vi "Simple QMH Template.vi"   [LabVIEW 2020, in "Volatus.lvlib"]
uses:
  Volatus.lvlib
  Module/Module.lvclass
types:
  T1 = enum32{"Invalid", "Standard", "Closed", "Hidden", "Minimized", "Maximized"}
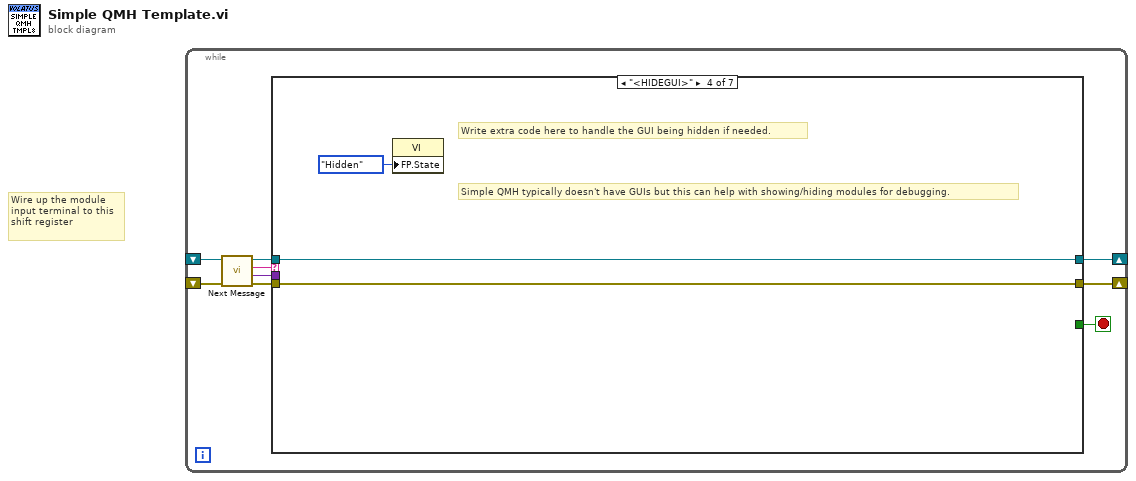
[diagram p0: block diagram]
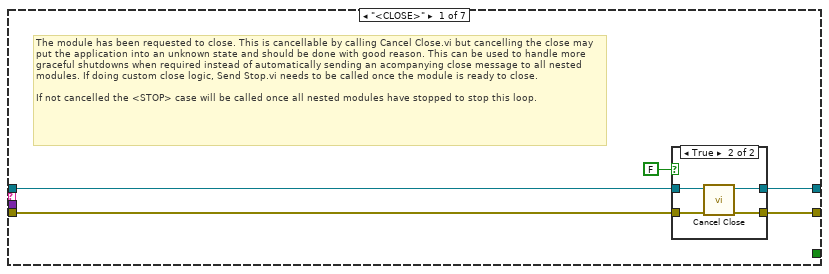
[diagram p2: hidden frame]
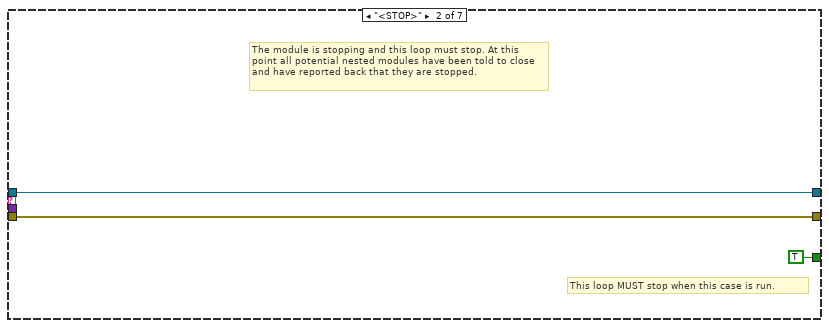
[diagram p4: hidden frame]
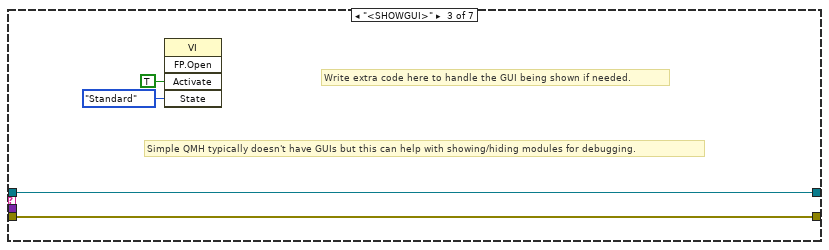
[diagram p5: hidden frame]
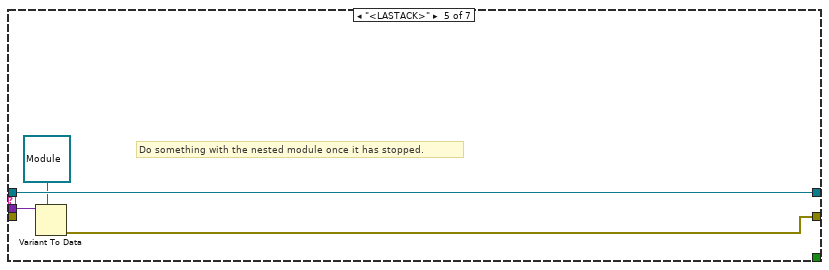
[diagram p6: hidden frame]
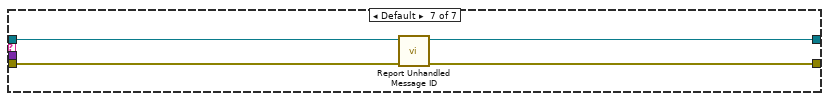
[diagram p8: hidden frame]
diagram:
  # "Wire up the module input terminal to this shift register"
  n1 = while {
    shift-right: [w4] -> _
    shift-left: _ -> [w9]
    shift-right: [w3] -> _
    shift-left: _ -> [w8]
    stop <- w2 stop-if-true
    n2 = call "Next Message.vi"("error in (no error)"=w8, "Module in"=w9) -> ("error out"=w7:errorcluster, "Data"=w1:variant, "ID"=w6:string, "Module out"=w5:refnum<class "Module.lvclass">)  [unwired: 6 in]
    n3 = case shown="\"<HIDEGUI>\"" w6 {
      tunnel: w7 -> [w14 w22 w26 w29 _ w35 w40]
      tunnel: w5 -> [w12 w23 w27 w30 w34 w36 w38]
      tunnel: [w11 w23 w27 w30 w34 w36 w37] -> w4
      tunnel: [w13 w22 w26 w29 w31 w35 w39] -> w3
      tunnel: [_ TRUE _ _ _ _ _] -> w2
      tunnel: w1 -> [_ _ _ _ w33 _ _]
      frame "<CLOSE>" {
        # "The module has been requested to close. This is cancellable by calling Cancel Close.vi but cancelling the close may put the application into an unknown state and should be done with good reason. This can be used to handle more graceful shutdowns when required instead of automatically sending an acompanying close message to all nested modules. If doing custom close logic, Send Stop.vi needs to be called once the module is ready to close.\n\nIf not cancelled the <STOP> case will be called once all nested modules have stopped to stop this loop."
        n4 = case shown="True" FALSE {
          tunnel: w14 -> [w15 w20]
          tunnel: [w15 w19] -> w13
          tunnel: w12 -> [w16 w18]
          tunnel: [w16 w17] -> w11
          frame False {
          }
          frame True {
            n5 = call "Cancel Close.vi"("error in (no error)"=w20, "Module in"=w18) -> ("error out"=w19:errorcluster, "Module out"=w17:refnum<class "Module.lvclass">)  [unwired: 8 in]
          }
        }
      }
      frame "<STOP>" {
        # "This loop MUST stop when this case is run."
        # "The module is stopping and this loop must stop. At this point all potential nested modules have been told to close and have reported back that they are stopped."
      }
      frame "<SHOWGUI>" {
        # "Simple QMH typically doesn't have GUIs but this can help with showing/hiding modules for debugging."
        # "Write extra code here to handle the GUI being shown if needed."
        n6 = invoke class="VI" method="FP.Open"("Activate"=TRUE ("Activate?"), "State"=T1."Standard") -> ()  [unwired: 3 in, 5 out]
      }
      frame "<HIDEGUI>" {
        # "Simple QMH typically doesn't have GUIs but this can help with showing/hiding modules for debugging."
        # "Write extra code here to handle the GUI being hidden if needed."
        n7 = property class="VI"("FP.State"=T1."Hidden" ("Front Panel Window:State")) -> ()  [unwired: 2 in, 2 out]
      }
      frame "<LASTACK>" {
        # "Do something with the nested module once it has stopped."
        n8 = Variant To Data(type=refnum<class "Module.lvclass"> refnum ("Volatus:Module"), Variant=w33) -> (error out=w31:errorcluster)  [unwired: 1 in, 1 out]
      }
      frame "<TIMEOUT>" {
        # "No message for this module was received in time"
      }
      frame Default {
        n9 = call "Report Unhandled Message ID.vi"("error in (no error)"=w40, "Module in"=w38) -> ("error out"=w39:errorcluster, "Module out"=w37:refnum<class "Module.lvclass">)  [unwired: 8 in]
      }
    }
  }
